vi "GetLeCroyPrams.vi"(11 "VISA session":refnum<visa-resource-name>) -> (0 "Waveform Graph":T1(graph), 1 "RF PTS":i32, 2 "Delay (micros)":dbl format="%.2f", 3 "Sampling Rate":u16(ring)=5, 4 "sampling time":sgl format="%.2f", 5 "RF Gain dB":sgl format="%.2f", 6 "TIMEBASE":i16)   [LabVIEW 2022 SP3]
panel:
  out "TRIGGER_TIME":dbl format="%.2f"
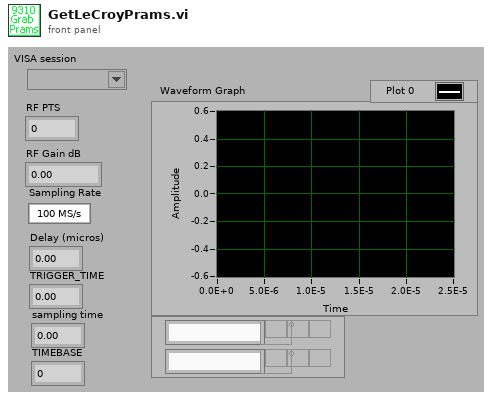
[diagram p1: front panel]
types:
  T1 = cluster{"t(0) (sec)":ext, "Delta t (sec)":dbl, "Amplitude Array (Volts)":sgl[]}
  T2 = cluster{"DESCRIPTOR_NAME":string, "TEMPLATE_NAME":string, "COMM_TYPE":i16, "COMM_ORDER":i16, "WAVE_DESCRIPTOR":i32, "USER_TEXT Leng":i32, "TRIGTIME_ARRAY Leng":i32, "RIS_TIME_ARRAY Leng":i32, "WAVE_ARRAY_1  Leng":i32, "WAVE_ARRAY_2  Leng":i32}
  T3 = cluster{"SUBARRAY_COUNT":i32, "SWEEPS_PER_ACQ":i32, "POINTS_PER_PAIR":i16, "PAIR_OFFSET":i16, "VERTICAL_GAIN":sgl, "VERTICAL_OFFSET":sgl, "MAX_VALUE":sgl, "MIN_VALUE":sgl, "NOMINAL_BITS":i16, "NOM_SUBAR_CNT":i16}
  T4 = cluster{"TIMEBASE":i16, "VERT_COUPLING":i16, "PROBE_ATT":sgl, "FIXED_VERT_GAIN":i16, "BANDWIDTH_LIM":i16, "VERTICAL_VERN":sgl, "ACQ_VERT_OFFS":sgl, "WAVE_SOURCE":i16}
  T5 = cluster{"HORIZ_INTERVAL":sgl, "HORIZ_OFFSET":dbl, "PIXEL_OFFSET":dbl, "VERTUNIT":string, "HORUNIT":string, "TRIGGER_TIME":dbl, "ACQ_DURATION":sgl, "RECORD_TYPE":i32, "PROCESS_DONE":i32, "RIS_SWEEPS":i32}
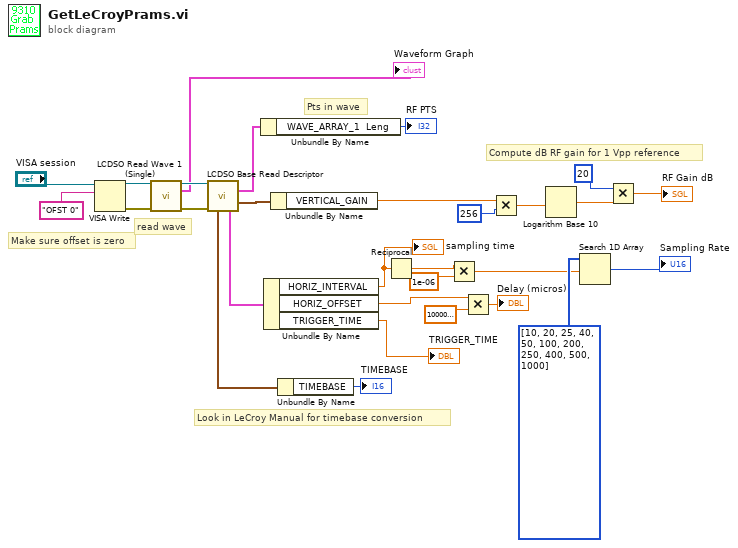
[diagram p0: block diagram]
diagram:
  # "Pts in wave"
  # "Compute dB RF gain for 1 Vpp reference"
  # "Look in LeCroy Manual for timebase conversion"
  # "read wave"
  # "Make sure offset is zero"
  n1 = VISA Write(VISA resource name="VISA session", write buffer="OFST 0") -> (VISA resource name out=w4:refnum<visa-resource-name>, error out=w2:errorcluster)  [unwired: 1 in, 1 out]
  n2 = call "LCDSO Read Wave 1 (Single).vi"("VISA session"=w4, "error in (no error)"=w2) -> ("dup VISA session"=w29:refnum<visa-resource-name>, "Wave Output"=→"Waveform Graph":T1, "error out"=w28:errorcluster)  [unwired: 8 in, 3 out]
  n3 = call "LCDSO Base Read Descriptor.vi"("VISA session"=w29, "error in (no error)"=w28) -> ("Parameters 1"=w22:T2, "Parameters 3"=w27:T3, "Parameters 5"=w9:T4, "Parameters 4"=w26:T5)  [unwired: 7 in, 3 out]
  n4 = Unbundle By Name(w22) -> ("WAVE_ARRAY_1  Leng"=→"RF PTS":i32)
  n5 = Unbundle By Name(w26) -> ("HORIZ_INTERVAL"=w24:sgl, "HORIZ_OFFSET"=w20:dbl, "TRIGGER_TIME"=→"TRIGGER_TIME":dbl)
  "sampling time" <- w24
  n6 = Unbundle By Name(w27) -> ("VERTICAL_GAIN"=w15:sgl)
  n7 = Unbundle By Name(w9) -> ("TIMEBASE"=→"TIMEBASE":i16)
  n8 = Reciprocal(x=w24) -> (1/x=w16:sgl)
  n9 = Multiply(x=w16, y=1e-06) -> (x*y=w5:dbl)
  n10 = Multiply(x=w20, y=1000000.0) -> (x*y=→"Delay (micros)":dbl)
  n11 = Multiply(x=w15, y=256) -> (x*y=w13:sgl)
  n12 = Logarithm Base 10(1:w13) -> (0:w12:sgl)
  n13 = Search 1D Array(1D array=i32[] [10, 20, 25, 40, 50, 100, 200, 250, 400, 500, 1000], element=w5) -> (index of element=→"Sampling Rate":i32)  [unwired: 1 in]
  n14 = Multiply(x=20, y=w12) -> (x*y=→"RF Gain dB":sgl)
